vi "Init.vi"(8 "error in (no error)":errorcluster, 10 "IConfigure in":refnum<class "IConfigure.lvclass">, 11 "IFGEN in":refnum<class "IFGEN.lvclass">) -> (0 "error out":errorcluster, 3 "IFGEN out":refnum<class "IFGEN.lvclass">)   [LabVIEW 2023, in "IFGEN.lvclass"]
uses:
  IFGEN.lvclass
  IConfigure/IConfigure.lvclass
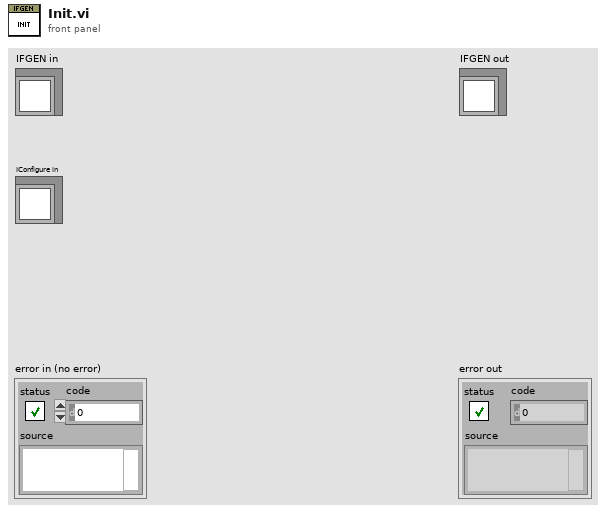
[diagram p1: front panel]
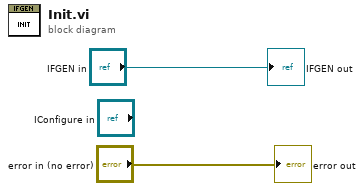
[diagram p0: block diagram]
diagram:
  "error out" <- "error in (no error)"
  "IFGEN out" <- "IFGEN in"
